vi "PathPlanner_PathFinder_FindClosestNonObstacle.vi"(11 "GridPosition":T1) -> (1 "Found":bool, 3 "NonObstacleGridPositin":T1)   [LabVIEW 2019, in "PathPlanner24.lvlib"]
uses:
  PathPlanner24.lvlib
  PathPlanner_PathFinder_Globals.vi
  TypeDef/PathPlannerFinderGridPosition.ctl
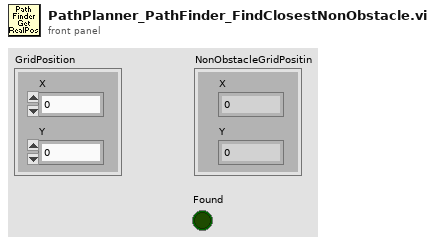
[diagram p1: front panel]
types:
  T1 = typedef "PathPlanner24.lvlib/PathPlannerFinderGridPosition.ctl" = cluster{"X":i32, "Y":i32}
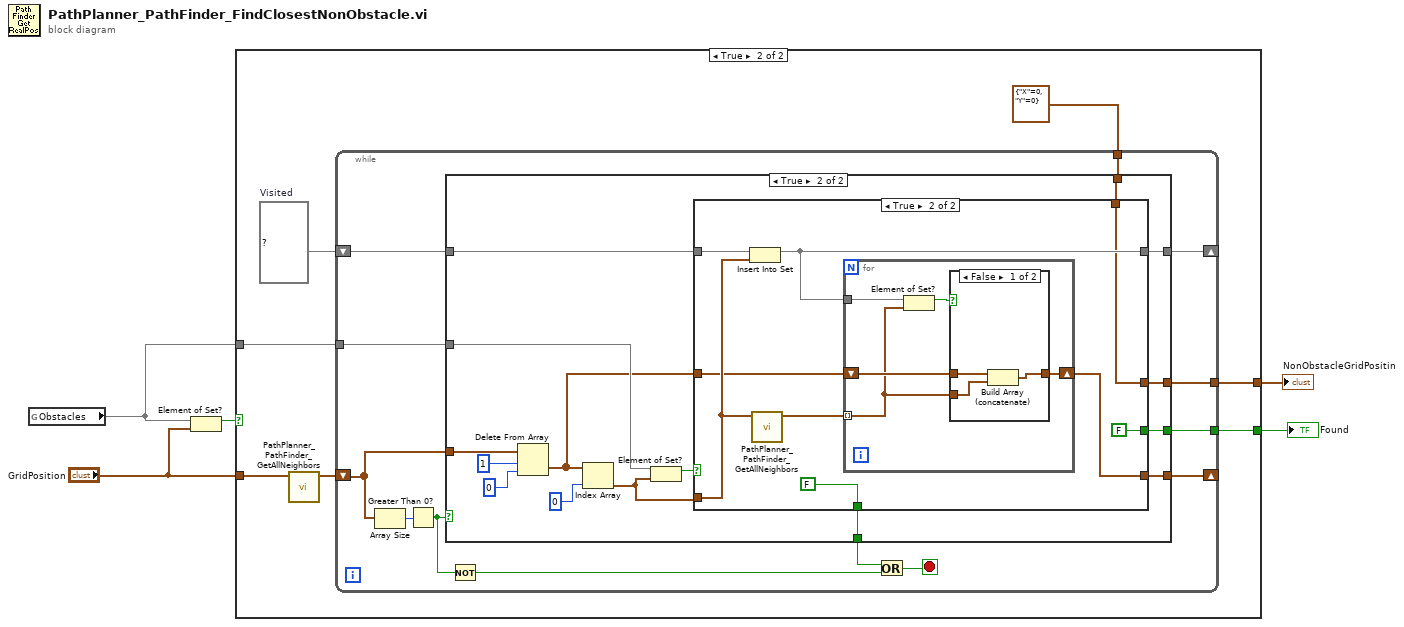
[diagram p0: block diagram]
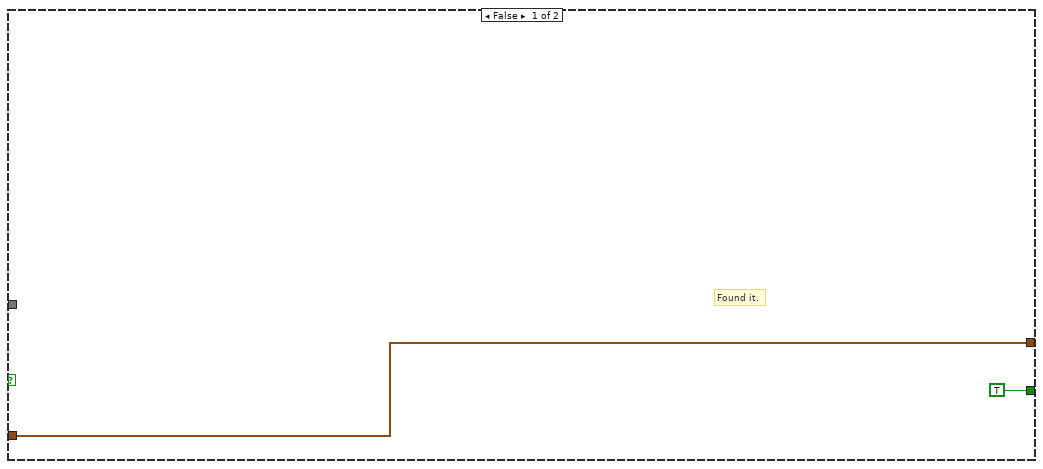
[diagram p2: hidden frame]
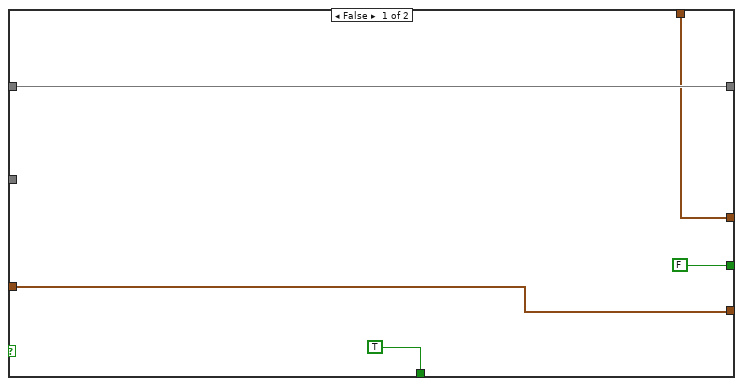
[diagram p3: hidden frame]
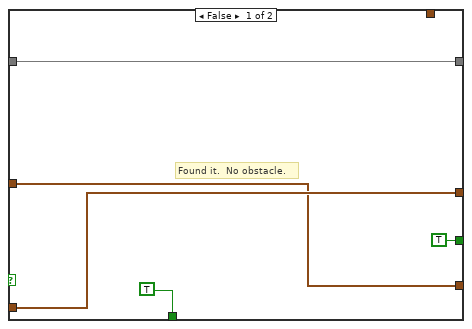
[diagram p4: hidden frame]
diagram:
  n1 = global read "PathPlanner_PathFinder_Globals.vi" "Obstacles"() -> (w2:set{T1})
  n2 = Element of Set?(10:"GridPosition", 11:w2) -> (3:w5:bool)
  n3 = case shown="True" w5 {
    tunnel: "GridPosition" -> [w7 w14]
    tunnel: [w7 w11] -> w3
    tunnel: w2 -> [_ w12]
    tunnel: [TRUE ("Found") w9] -> w1
    frame False {
      # "Found it."
    }
    frame True {
      w10 = set{T1} {}  # Visited
      n4 = call "PathPlanner_PathFinder_GetAllNeighbors.vi"("GridPosition"=w14) -> ("Neighbors"=w13:T1[])  [unwired: 10 in]
      n5 = while {
        shift-right: [w17] -> _
        shift-left: w13 -> [w22]
        tunnel: w12 -> [w21]
        tunnel: [w20] -> w11
        shift-right: [w18] -> _
        shift-left: w10 -> [w19]
        tunnel: [w16] -> w9
        tunnel: T1 {"X"=0, "Y"=0} ("Neighbors") -> [w15]
        stop <- w25 stop-if-true
        n6 = Array Size(array=w22) -> (size(s)=w27:i32)
        n7 = Greater Than 0?(x=w27) -> (x > 0?=w26:bool)
        n8 = case shown="True" w26 {
          tunnel: [TRUE w42] -> w23
          tunnel: w22 -> [w29 w38]
          tunnel: w21 -> [_ w44]
          tunnel: [w28 w41] -> w20
          tunnel: w19 -> [w31 w39]
          tunnel: [w31 w37] -> w18
          tunnel: [w29 w36] -> w17
          tunnel: [FALSE w35] -> w16
          tunnel: w15 -> [w28 w34]
          frame False {
          }
          frame True {
            n9 = Delete From Array(array=w38, length=1, index=0) -> (deleted portion=w33:T1[])  [unwired: 1 out]
            n10 = Index Array(array=w33, index=0) -> (element=w40:T1)
            n11 = Element of Set?(10:w40, 11:w44) -> (3:w43:bool)
            n12 = case shown="True" w43 {
              tunnel: [TRUE FALSE] -> w42
              tunnel: [w51 w53] -> w41
              tunnel: w40 -> [w51 w59]
              tunnel: w39 -> [w49 w60]
              tunnel: w33 -> [w50 w57]
              tunnel: [w49 w56] -> w37
              tunnel: [w50 w55] -> w36
              tunnel: [TRUE FALSE] -> w35
              tunnel: w34 -> [_ w53]
              frame False {
                # "Found it.  No obstacle."
              }
              frame True {
                n13 = Insert Into Set(10:w59, 11:w60) -> (3:w56:set{T1})  [unwired: 1 out]
                n14 = call "PathPlanner_PathFinder_GetAllNeighbors.vi"("GridPosition"=w59) -> ("Neighbors"=w58:T1[])  [unwired: 10 in]
                n15 = for {
                  tunnel: w58 -> [w62] mode=indexing
                  shift-right: [w63] -> w55
                  shift-left: w57 -> [w64]
                  tunnel: w56 -> [w66]
                  n16 = Element of Set?(10:w62, 11:w66) -> (3:w65:bool)
                  n17 = case shown="False" w65 {
                    tunnel: w64 -> [w69 w70]
                    tunnel: [w67 w70] -> w63
                    tunnel: w62 -> [w68 _]
                    frame False {
                      n18 = Build Array (concatenate)(w69, w68) -> (w67:T1[])
                    }
                    frame True {
                    }
                  }
                }
              }
            }
          }
        }
        n19 = Not(x=w26) -> (.not. x?=w24:bool)
        n20 = Or(x=w23, y=w24) -> (x .or. y?=w25:bool)
      }
    }
  }
  "NonObstacleGridPositin" <- w3
  "Found" <- w1
